vi "func-YtStringPath2legal.vi"(10 "change char( _ )":string="_", 11 "StringPath in":string) -> (3 "StringPath out":string)   [LabVIEW 2017]
panel:
  # "This for Step vi"
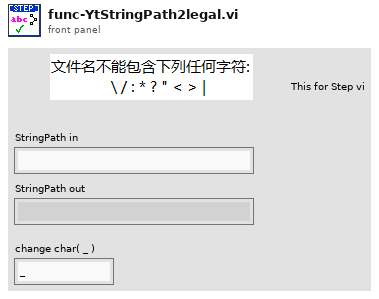
[diagram p1: front panel]
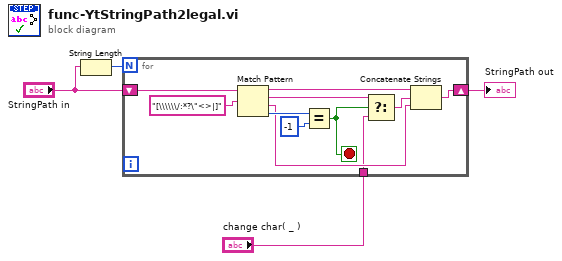
[diagram p0: block diagram]
diagram:
  n1 = String Length(string="StringPath in") -> (length=w2:i32)
  n2 = for {
    N: w2 -> [_]
    shift-right: [w7] -> w4
    shift-left: "StringPath in" -> [w15]
    tunnel: "change char( _ )" -> [w5]
    stop <- w6 stop-if-true
    n3 = Match Pattern(string=w15, regular expression="[\\\\\\/:*?\"<>|]") -> (before substring=w11:string, match substring=w8:string, after substring=w9:string, offset past match=w13:i32)  [unwired: 1 in]
    n4 = Equal?(x=w13, y=-1) -> (x = y?=w6:bool)
    n5 = Select(t=w8, s=w6, f=w5) -> (s? t:f=w10:string)
    n6 = Concatenate Strings(w11, w10, w9) -> (w7:string)
  }
  "StringPath out" <- w4
